vi "Export.vi"(8 "error in (no error)":errorcluster, 11 "JUnit for Azure Pipelines in":refnum<class "JUnit for Azure Pipelines.lvclass">) -> (0 "error out":errorcluster, 3 "JUnit for Azure Pipelines out":refnum<class "JUnit for Azure Pipelines.lvclass">)   [LabVIEW 2013, in "JUnit for Azure Pipelines.lvclass"]
uses:
  JUnit for Azure Pipelines.lvclass
  JUnit for Azure Pipelines.lvclass/JUnit for Azure Pipelines.ctl
  <vilib>/addons/_JKI Toolkits/Caraya/classes/Test Report/Test Report.lvclass/Test Report.ctl
  <vilib>/PNR/JUnit XML/JUnit XML/Test Suites/Test Suites.lvclass
  <vilib>/addons/_JKI Toolkits/Caraya/classes/Test Report/Test Report.lvclass
  <vilib>/addons/_JKI Toolkits/Caraya/classes/Test Result/Test Result.lvclass
  JUnit Conversion/JUnit Conversion.lvlib
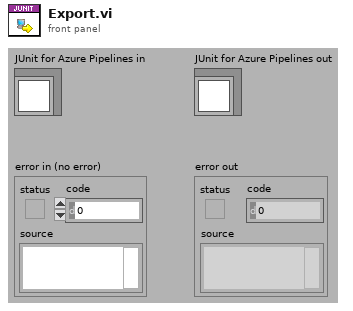
[diagram p1: front panel]
types:
  T1 = typedef "Caraya.lvlib/Test Result.lvclass/Node Results (Extended).ctl" = cluster{"Test Node":T2, "Assertions":T4[]}
  T2 = typedef "Caraya.lvlib/Test Result.lvclass/Test Node (Extended).ctl" = cluster{"Test Registration":T3, "Defined":bool, "Passed":bool, "properties":variant}
  T3 = typedef "Caraya.lvlib/Test Result.lvclass/Test Registration Data.ctl" = cluster{"Name":string, "Call Chain":string[], "Time Stamp":timestamp, "Test ID":string, "Caller ID":string}
  T4 = typedef "Caraya.lvlib/Test Result.lvclass/Assert Event Data (Extended).ctl" = cluster{"name":string, "passed":bool, "call-chain":string[], "test-error":errorcluster, "timestamp":timestamp, "assert-id":string, "test-id":string, "time":dbl, "message":string, "properties":variant, "measurements":variant, "user-defined":variant}
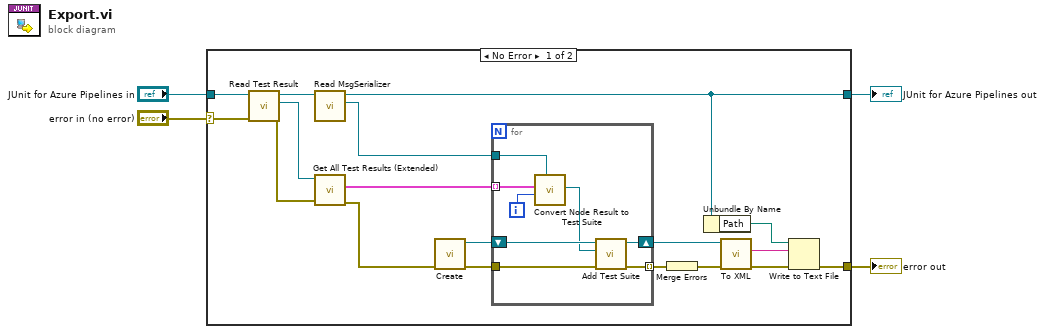
[diagram p0: block diagram]
diagram:
  n1 = case shown="No Error" "error in (no error)" {
    selector: "error in (no error)" -> [w21 w31]
    tunnel: [w6 w31] -> w3
    tunnel: "JUnit for Azure Pipelines in" -> [w22 w32]
    tunnel: [w16 w32] -> w1
    frame No Error {
      n2 = call <vilib>:"Read Test Result.vi"("error in (no error)"=w21, "Test Report in"=w22) -> ("error out"=w20:errorcluster, "Caraya.lvlib:Test Result.lvclass"=w19:refnum<class "Test Result.lvclass">, "Test Report out"=w17:refnum<class "JUnit for Azure Pipelines.lvclass">)  [unwired: 7 in]
      n3 = call <vilib>:"Read MsgSerializer.vi"("Test Report in"=w17) -> ("MsgSerializer"=w15:refnum<class "MsgSerializer.lvclass">, "Test Report out"=w16:refnum<class "JUnit for Azure Pipelines.lvclass">)  [unwired: 9 in]
      n4 = call <vilib>:"Get All Test Results (Extended).vi"("error in (no error)"=w20, "Test Result in"=w19) -> ("error out"=w13:errorcluster, "Test Results"=w14:T1[])  [unwired: 7 in, 1 out]
      n5 = call <vilib>:"Create.vi"("error in (no error)"=w13) -> ("error out"=w12:errorcluster, "Test Suites"=w10:refnum<class "Test Suites.lvclass">)  [unwired: 9 in]
      n6 = for {
        tunnel: w14 -> [w26] mode=indexing
        tunnel: [w29] -> w18 mode=indexing
        tunnel: w12 -> [w30]
        shift-right: [w27] -> w8
        shift-left: w10 -> [w28]
        tunnel: w15 -> [w24]
        i -> [w25]
        n7 = call "Convert Node Result to Test Suite.vi"("MsgSerializer"=w24, "ID"=w25, "Node Result"=w26) -> ("Test Suite"=w23:refnum<class "Test Suite.lvclass">)  [unwired: 8 in]
        n8 = call <vilib>:"Add Test Suite.vi"("error in (no error)"=w30, "Test Suite"=w23, "Test Suites in"=w28) -> ("error out"=w29:errorcluster, "Test Suites out"=w27:refnum<class "Test Suites.lvclass">)  [unwired: 7 in]
      }
      n9 = Merge Errors(w18) -> (w11:errorcluster)
      n10 = Unbundle By Name(w16) -> ("Path"=w7:path)
      n11 = call-dynamic "To XML.vi"("error in (no error)"=w11, "Serializable in"=w8) -> ("error out"=w9:errorcluster, "XML"=w5:string)  [unwired: 8 in]
      n12 = Write to Text File(file (use dialog)=w7, text=w5, error in=w9) -> (error out=w6:errorcluster)  [unwired: 1 in, 2 out]
    }
    frame Error {
    }
  }
  "error out" <- w3
  "JUnit for Azure Pipelines out" <- w1
